vi "Fdx Create Rx VL.vi"(8 "error in (no error)":errorcluster, 10 "VL Config":T1={"VlId"=1, "VLRange"=1, "VerificationMode"=0, "Bag"=0, "Jitter"=0, "MaxFrameLength"=0, "MaxSkew"=0, "VLBufSize"=32768, "FilterMode"=0, "FilterPosition"=0, "Padding"=0, "FilterMask"=0, "FilterData"=0, "MinFrameLength"=0} {"FilterMode" items=["FDX_RX_VL_FLT_DIS", "FDX_RX_VL_FLT_ENA ", "FDX_RX_VL_FLT_ENA_INV"]; "MaxFrameLength" format="%.0x"; "VerificationMode" items=["FDX_RX_VL_CHECK_ENA_DEFAULT"=65535, "FDX_RX_VL_CHECK_REDMAM"=16, "DX_RX_VL_CHECK_TRAFIC"=8, "FDX_RX_VL_CHECK_FRAMESIZE"=4, "FDX_RX_VL_CHECK_SNINTEG"=2, "FDX_RX_VL_CHECK_INVPAC"=1, "FDX_RX_VL_CHECK_DISA"=0]}, 11 "InstrumentHandle_port in":u32) -> (0 "error out":errorcluster, 1 "VlId":u16, 3 "InstrumentHandle_port out":u32)   [LabVIEW 2020, in "AIM664LV.lvlib"]
doc: "This function is used to control the Virtual link specific setting for a receive port.\n\n<B>VLRange</B>: Number of VLs which are affected by the TY_FDX_RX_VL_CTRL settings, beginning with the VL set in the ul_VLId parameter\n<B>TCBIndex</B>: This value defines the Trigger Control Block (TCB) Index \n\n<B>Bag</B>: Bandwidth Allocation Gap (BAG) for the defined Virtual Link.\nAs shown below, this parameter is interpreted differently depending on the value of Bit 31 (1- bag in uS, 0 - bag in mS)\n<B>Jitter</B>: maximum allowed jitter in uS\n<B>MaxFrameLenght (MinFrameLenght)</B>: Maximum/Minimum Frame Length of a MAC Frame specified for this Virtual Link.\n<B>VLBufSize</B>: If this value is set to 0, the onboard target software will set to a default value."
uses:
  AIM664LV.lvlib
  _controls/comm_verification_rx.ctl
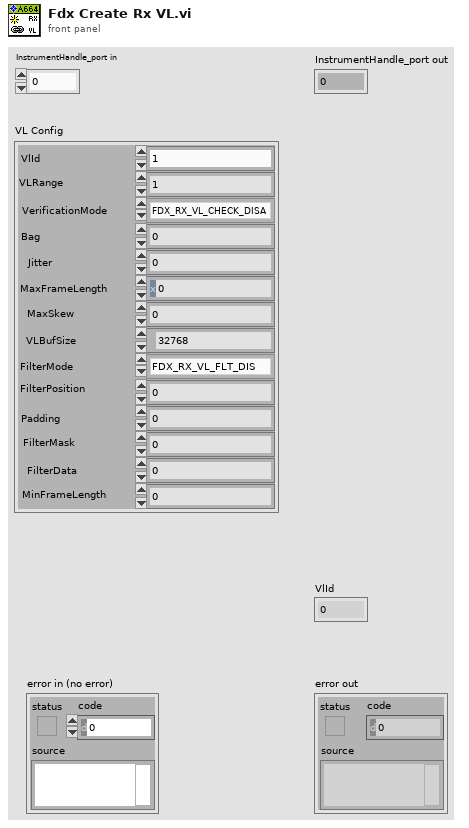
[diagram p1: front panel]
types:
  T1 = typedef "AIM664LV.lvlib/comm_verification_rx.ctl" = cluster{"VlId":u16, "VLRange":u32, "VerificationMode":u32, "Bag":u32, "Jitter":u32, "MaxFrameLength":u32, "MaxSkew":u32, "VLBufSize":u32, "FilterMode":u32, "FilterPosition":u32, "Padding":u32, "FilterMask":u32, "FilterData":u32, "MinFrameLength":u32}
  T2 = cluster{"VLId":u32, "VLRange":u32, "EnableMode":u32, "PayloadMode":u32, "TCBIndex":u32, "VerificationMode":u32, "Bag":u32, "Jitter":u32, "MaxFrameLength":u32, "MaxSkew":u32, "VLBufSize":u32, "FilterMode":u32, "FilterPosition":u32, "Padding":u32, "FilterMask":u32, "FilterData":u32, "MinFrameLength":u32}
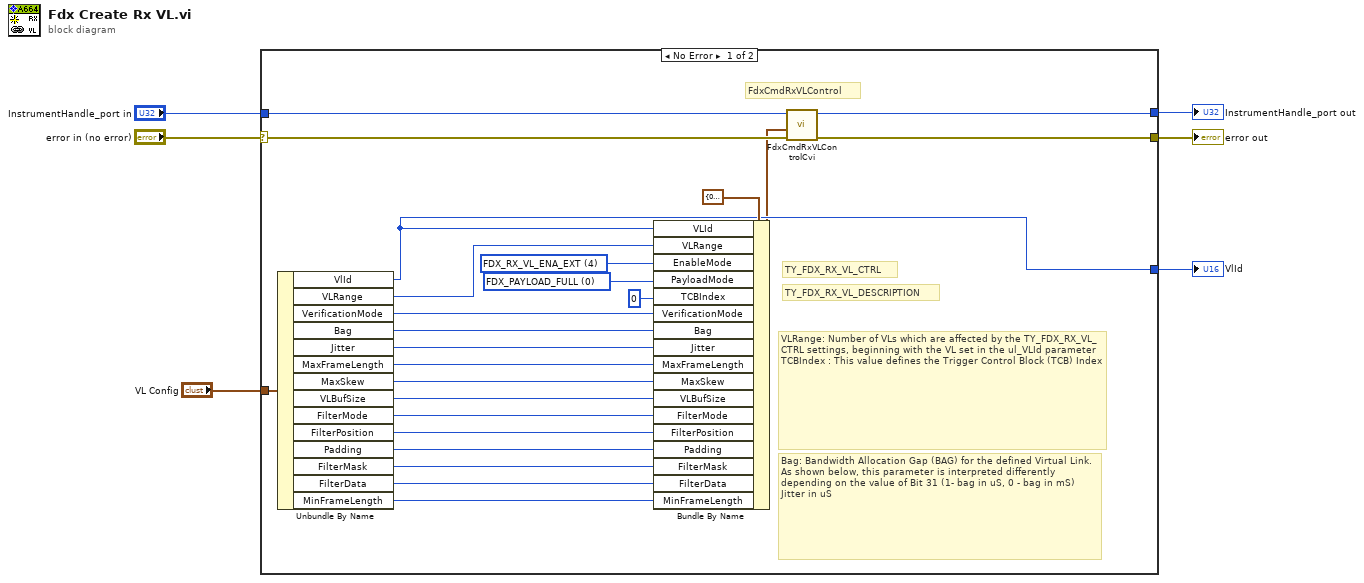
[diagram p0: block diagram]
diagram:
  n1 = case shown="No Error" "error in (no error)" {
    selector: "error in (no error)" -> [w29 w32]
    tunnel: [w30 w32] -> w5
    tunnel: [w8 w31] -> w3
    tunnel: "InstrumentHandle_port in" -> [w7 w31]
    tunnel: "VL Config" -> [w24 _]
    tunnel: [w10 _] -> w1
    frame No Error {
      w26 = u32 0 items=["FDX_PAYLOAD_FULL", "FDX_PAYLOAD_IP_EXT", "FDX_PAYLOAD_IP", "FDX_PAYLOAD_MAC"] ("PayloadMode")
      w27 = u32 4 items=["FDX_RX_VL_DIS "=0, "FDX_RX_VL_ENA_STAT"=1, "FDX_RX_VL_ENA_CNT "=2, "FDX_RX_VL_ENA_MON_ALL"=3, "FDX_RX_VL_ENA_MON_GOOD"=7, "FDX_RX_VL_ENA_EXT"=4] ("EnableMode")
      # "FdxCmdRxVLControl"
      # "Bag: Bandwidth Allocation Gap (BAG) for the defined Virtual Link.\nAs shown below, this parameter is interpreted differently depending on the value of Bit 31 (1- bag in uS, 0 - bag in mS)\nJitter in uS"
      # "TY_FDX_RX_VL_DESCRIPTION"
      # "TY_FDX_RX_VL_CTRL"
      # "VLRange: Number of VLs which are affected by the TY_FDX_RX_VL_CTRL settings, beginning with the VL set in the ul_VLId parameter\nTCBIndex : This value defines the Trigger Control Block (TCB) Index"
      n2 = Unbundle By Name(w24) -> ("VlId"=w10:u16, "VLRange"=w11:u32, "VerificationMode"=w12:u32, "Bag"=w13:u32, "Jitter"=w14:u32, "MaxFrameLength"=w15:u32, "MaxSkew"=w16:u32, "VLBufSize"=w17:u32, "FilterMode"=w18:u32, "FilterPosition"=w19:u32, "Padding"=w20:u32, "FilterMask"=w21:u32, "FilterData"=w22:u32, "MinFrameLength"=w23:u32)
      n3 = Bundle By Name(cluster=T2 {"VLId"=0, "VLRange"=0, "EnableMode"=0, "PayloadMode"=0, "TCBIndex"=0, "VerificationMode"=0, "Bag"=0, "Jitter"=0, "MaxFrameLength"=0, "MaxSkew"=0, "VLBufSize"=0, "FilterMode"=0, "FilterPosition"=0, "Padding"=0, "FilterMask"=0, "FilterData"=0, "MinFrameLength"=0} ("VLControl"), "VLId"=w10, "VLRange"=w11, "EnableMode"=w27, "PayloadMode"=w26, "TCBIndex"=u32 0, "VerificationMode"=w12, "Bag"=w13, "Jitter"=w14, "MaxFrameLength"=w15, "MaxSkew"=w16, "VLBufSize"=w17, "FilterMode"=w18, "FilterPosition"=w19, "Padding"=w20, "FilterMask"=w21, "FilterData"=w22, "MinFrameLength"=w23) -> (w9:T2)
      n4 = call "FdxCmdRxVLControlCvi.vi"("error in"=w29, "VLControl"=w9, "InstrumentHandle_port"=w7) -> ("error out"=w30:errorcluster, "InstrumentHandle_port"=w8:u32)  [unwired: 7 in]
    }
    frame Error {
    }
  }
  "error out" <- w5
  "InstrumentHandle_port out" <- w3
  "VlId" <- w1
